vi "Twist Angle.vi"(3 "Thickness":dbl=0.33 format="%#_13g", 4 "Thickness Measured":dbl=0.695, 5 "Width":dbl=1.8 format="%#_13g") -> (0 "Theta t (Degree)":dbl, 1 "String":string, 2 "Theta t":dbl)   [LabVIEW 2019, in "Algorithm.lvclass"]
uses:
  FrameworkOverrides/Algorithm.lvclass
panel:
  out "Root -":dbl
  out "Root +":dbl
  out "c":dbl
  out "b":dbl
  out "a":dbl
  in  "Theta c":dbl
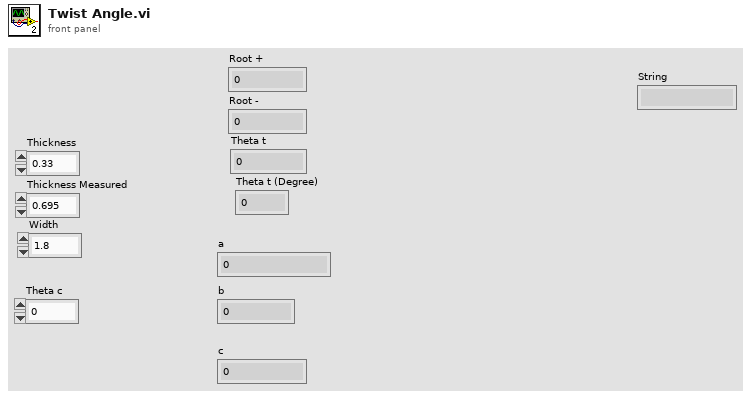
[diagram p1: front panel]
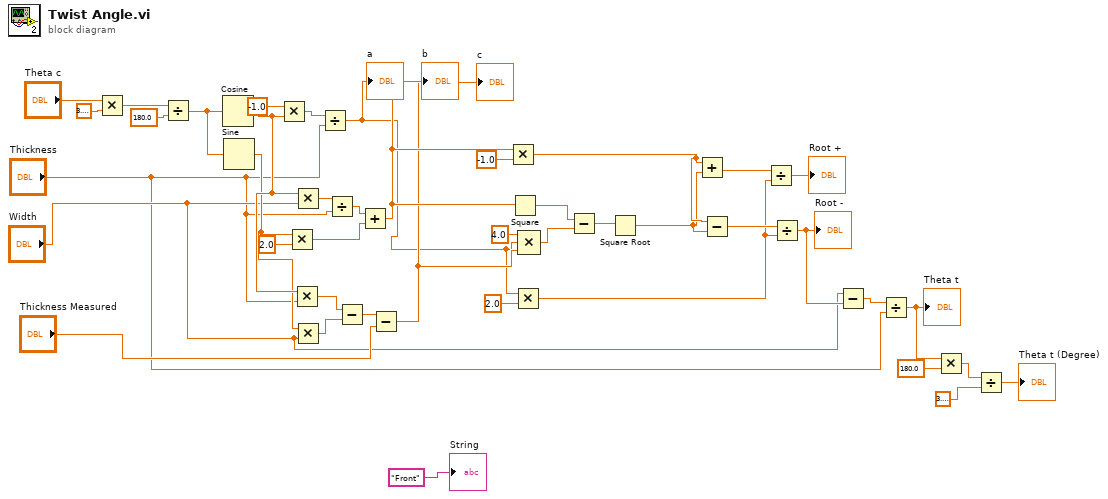
[diagram p0: block diagram]
diagram:
  n1 = Multiply(x="Theta c", y=3.141592653589793) -> (x*y=w41:dbl)
  n2 = Divide(x=w41, y=180.0) -> (x/y=w38:dbl)
  n3 = Cosine(x=w38) -> (cos(x)=w31:dbl)
  n4 = Sine(x=w38) -> (sin(x)=w30:dbl)
  n5 = Multiply(x=-1.0, y=w31) -> (x*y=w36:dbl)
  n6 = Multiply(x=w30, y=2.0) -> (x*y=w32:dbl)
  n7 = Multiply(x=w31, y="Thickness") -> (x*y=w29:dbl)
  n8 = Multiply(x=w31, y="Width") -> (x*y=w35:dbl)
  n9 = Multiply(x=w30, y="Width") -> (x*y=w28:dbl)
  n10 = Divide(x=w36, y="Thickness") -> (x/y=w17:dbl)
  "a" <- w17
  n11 = Divide(x=w35, y="Thickness") -> (x/y=w33:dbl)
  n12 = Subtract(x=w29, y=w28) -> (x-y=w27:dbl)
  n13 = Add(x=w33, y=w32) -> (x+y=w24:dbl)
  "b" <- w24
  n14 = Subtract(x=w27, y="Thickness Measured") -> (x-y=w22:dbl)
  "c" <- w22
  n15 = Multiply(x=w24, y=-1.0) -> (x*y=w16:dbl)
  n16 = Square(x=w24) -> (x^2=w21:dbl)
  n17 = Multiply(x=w17, y=2.0) -> (x*y=w12:dbl)
  n18 = Compound Arithmetic op=MULTIPLY(4.0 ("value"), w17, w22) -> (w20:dbl)
  n19 = Subtract(x=w21, y=w20) -> (x-y=w19:dbl)
  n20 = Square Root(x=w19) -> (sqrt(x)=w15:dbl)
  n21 = Add(x=w16, y=w15) -> (x+y=w14:dbl)
  n22 = Subtract(x=w16, y=w15) -> (x-y=w13:dbl)
  n23 = Divide(x=w14, y=w12) -> (x/y=→"Root +":dbl)
  n24 = Divide(x=w13, y=w12) -> (x/y=w10:dbl)
  "Root -" <- w10
  n25 = Subtract(x="Width", y=w10) -> (x-y=w8:dbl)
  n26 = Divide(x=w8, y="Thickness") -> (x/y=w6:dbl)
  "Theta t" <- w6
  n27 = Multiply(x=w6, y=180.0) -> (x*y=w4:dbl)
  n28 = Divide(x=w4, y=3.141592653589793) -> (x/y=→"Theta t (Degree)":dbl)
  "String" <- "Front"
